vi "Texte in VIs uebersetzen.vi"(0 "Sprachliste":string[][](array[string]), 5 "String-Array zum Übersetzen":string[](array[string]), 7 "2D String-Array zum Übersetzen":string[][](array[string]), 9 "String zum Übersetzen":string, 11 "error in (no error)":errorcluster caption="Fehler (Eingang, kein Fehler)") -> (4 "Sprachliste out":string[][](array[string]), 6 "String-Array zum Übersetzen":string[](array[string]), 8 "2D String-Array zum Übersetzen":string[][](array[string]), 10 "String zum Übersetzen":string, 15 "error out":errorcluster caption="Fehler (Ausgang)")   [LabVIEW 2020, in "Sprachverwaltung.lvlib"]
uses:
  Sprachverwaltung.lvlib
  Seiten/System Einstellungen V2/System Einstellungen V2.lvlib
  Seiten/System Einstellungen V2/Aktioen FGV System Konstanten.ctl
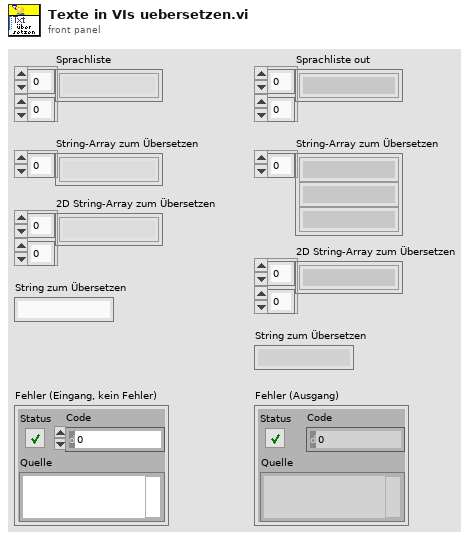
[diagram p1: front panel]
types:
  T1 = typedef "System Einstellungen V2.lvlib/Aktioen FGV System Konstanten.ctl" = enum16{"lesen", "laden", "speichern", "Sprache"}
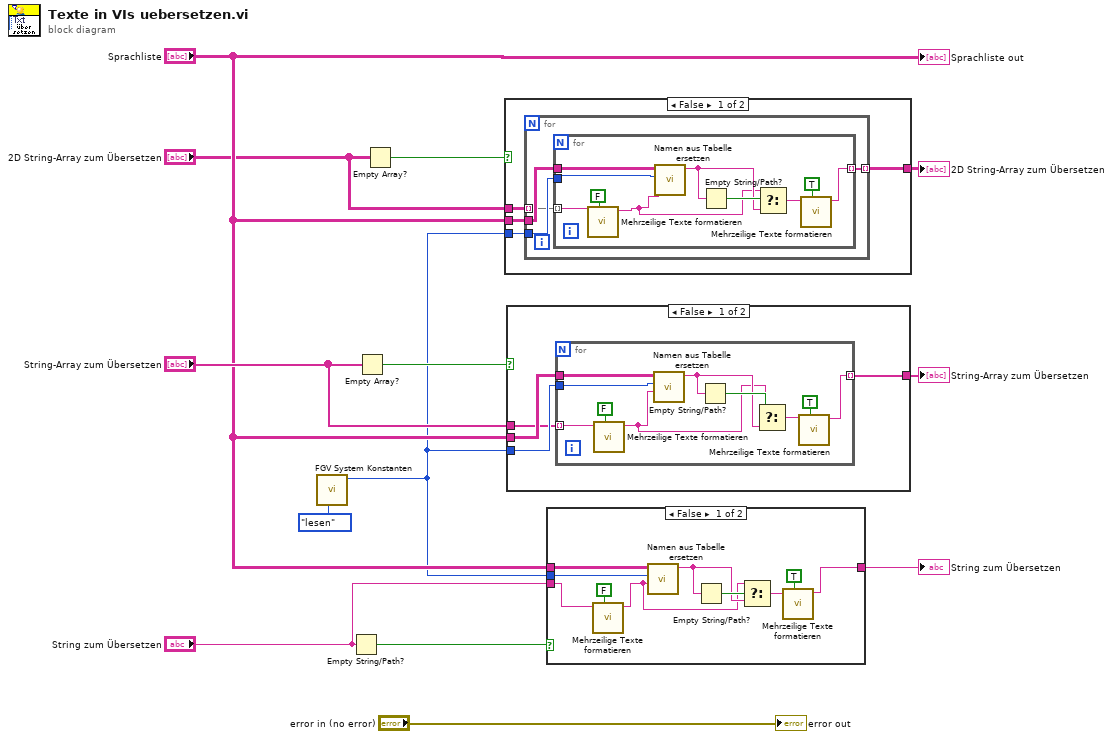
[diagram p0: block diagram]
diagram:
  n1 = call "FGV System Konstanten.vi"("Aktionen"=Aktioen_FGV_System_Konstanten."lesen") -> ("Sprachindex"=w1:u16)  [unwired: 6 in, 4 out]
  n2 = Empty String/Path?(string/path="String zum Übersetzen") -> (empty?=w12:bool)
  n3 = Empty Array?(array="String-Array zum Übersetzen") -> (empty?=w7:bool)
  n4 = Empty Array?(array="2D String-Array zum Übersetzen") -> (empty?=w5:bool)
  n5 = case shown="False" w5 {
    tunnel: "Sprachliste" -> [w17 _]
    tunnel: w1 -> [w16 _]
    tunnel: [w15 w32] -> w2
    tunnel: "2D String-Array zum Übersetzen" -> [w14 w32]
    frame False {
      n6 = for {
        tunnel: w17 -> [w21]
        tunnel: w16 -> [w20]
        tunnel: [w19] -> w15 mode=indexing
        tunnel: w14 -> [w18] mode=indexing
        n7 = for {
          tunnel: w21 -> [w31]
          tunnel: w20 -> [w30]
          tunnel: [w22] -> w19 mode=indexing
          tunnel: w18 -> [w26] mode=indexing
          n8 = call "Mehrzeilige Texte formatieren.vi"("Zurück formatieren"=FALSE, "string"=w26) -> ("result string"=w25:string)  [unwired: 9 in]
          n9 = call "Namen aus Tabelle ersetzen.vi"("Regulärer Ausdruck"=w25, "Sprachauswahl"=w30, "Tabelle"=w31) -> ("Übersetzung"=w28:string)  [unwired: 8 in]
          n10 = Empty String/Path?(string/path=w28) -> (empty?=w29:bool)
          n11 = Select(t=w25, s=w29, f=w28) -> (s? t:f=w23:string)
          n12 = call "Mehrzeilige Texte formatieren.vi"("Zurück formatieren"=TRUE, "string"=w23) -> ("result string"=w22:string)  [unwired: 9 in]
        }
      }
    }
    frame True {
    }
  }
  "2D String-Array zum Übersetzen" <- w2
  n13 = case shown="False" w7 {
    tunnel: "Sprachliste" -> [w36 _]
    tunnel: w1 -> [w35 _]
    tunnel: [w34 w47] -> w10
    tunnel: "String-Array zum Übersetzen" -> [w33 w47]
    frame False {
      n14 = for {
        tunnel: w36 -> [w46]
        tunnel: w35 -> [w45]
        tunnel: [w37] -> w34 mode=indexing
        tunnel: w33 -> [w41] mode=indexing
        n15 = call "Mehrzeilige Texte formatieren.vi"("Zurück formatieren"=FALSE, "string"=w41) -> ("result string"=w40:string)  [unwired: 9 in]
        n16 = call "Namen aus Tabelle ersetzen.vi"("Regulärer Ausdruck"=w40, "Sprachauswahl"=w45, "Tabelle"=w46) -> ("Übersetzung"=w43:string)  [unwired: 8 in]
        n17 = Empty String/Path?(string/path=w43) -> (empty?=w44:bool)
        n18 = Select(t=w40, s=w44, f=w43) -> (s? t:f=w38:string)
        n19 = call "Mehrzeilige Texte formatieren.vi"("Zurück formatieren"=TRUE, "string"=w38) -> ("result string"=w37:string)  [unwired: 9 in]
      }
    }
    frame True {
    }
  }
  "String-Array zum Übersetzen" <- w10
  n20 = case shown="False" w12 {
    tunnel: "Sprachliste" -> [w57 _]
    tunnel: w1 -> [w56 _]
    tunnel: "String zum Übersetzen" -> [w52 w58]
    tunnel: [w48 w58] -> w9
    frame False {
      n21 = call "Mehrzeilige Texte formatieren.vi"("Zurück formatieren"=FALSE, "string"=w52) -> ("result string"=w51:string)  [unwired: 9 in]
      n22 = call "Namen aus Tabelle ersetzen.vi"("Regulärer Ausdruck"=w51, "Sprachauswahl"=w56, "Tabelle"=w57) -> ("Übersetzung"=w54:string)  [unwired: 8 in]
      n23 = Empty String/Path?(string/path=w54) -> (empty?=w55:bool)
      n24 = Select(t=w51, s=w55, f=w54) -> (s? t:f=w49:string)
      n25 = call "Mehrzeilige Texte formatieren.vi"("Zurück formatieren"=TRUE, "string"=w49) -> ("result string"=w48:string)  [unwired: 9 in]
    }
    frame True {
    }
  }
  "String zum Übersetzen" <- w9
  "error out" <- "error in (no error)"
  "Sprachliste out" <- "Sprachliste"
